vi "Handle getAll.vi"(8 "error in (no error)":errorcluster, 11 "Instrument in":refnum<class "Instrument.lvclass">) -> (0 "error out":errorcluster, 2 "getAll":variant, 3 "Instrument out":refnum<class "Instrument.lvclass">)   [LabVIEW 2019, in "Instrument.lvlib" / "Instrument.lvclass"]
doc: "Override to handle \"getAll\" or \"getAllData\" commands for <b>your</b> Instrument"
uses:
  Instrument.lvclass
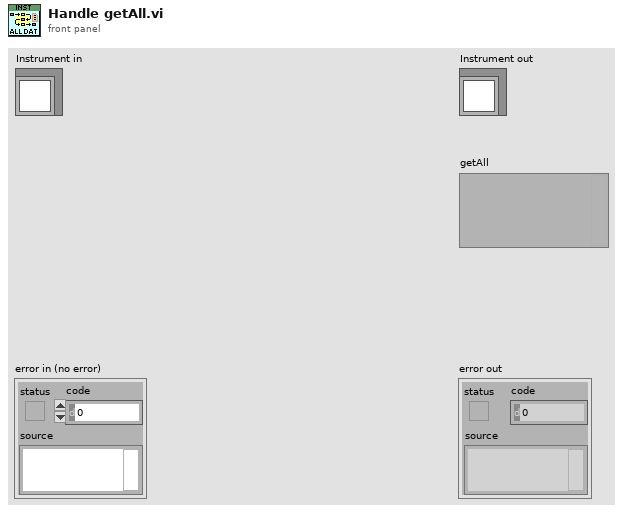
[diagram p1: front panel]
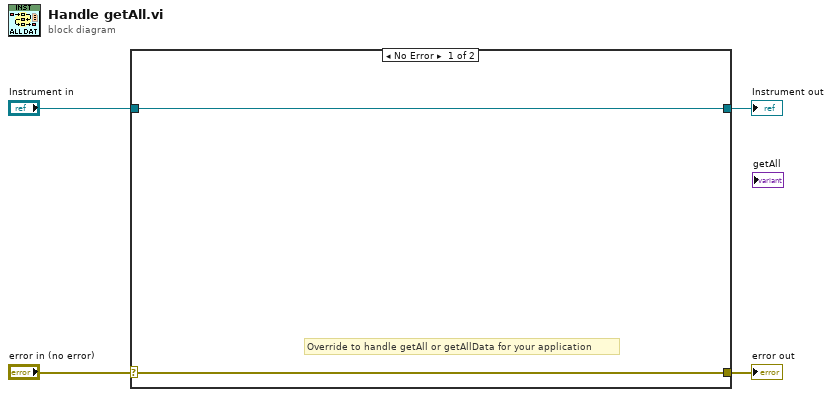
[diagram p0: block diagram]
diagram:
  n1 = case shown="No Error" "error in (no error)" {
    selector: "error in (no error)" -> [w6 w8]
    tunnel: [w6 w8] -> w3
    tunnel: [w5 w7] -> w1
    tunnel: "Instrument in" -> [w5 w7]
    frame No Error {
      # "Override to handle getAll or getAllData for your application"
    }
    frame Error {
    }
  }
  "error out" <- w3
  "Instrument out" <- w1
